vi "Get Value.vi"(10 "Key":string, 11 "Object Entry in":refnum<class "Section.lvclass">) -> (1 "Found?":bool, 2 "Value":refnum<class "Value.lvclass">, 3 "Object Entry out":refnum<class "Section.lvclass">)   [LabVIEW 2024, in "Electronic Datasheet.lvlib" / "Section.lvclass"]
uses:
  Section.lvclass
  Value/Value.lvclass
  Section.lvclass/Section.ctl
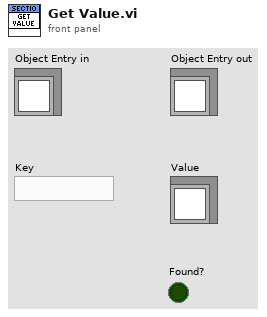
[diagram p1: front panel]
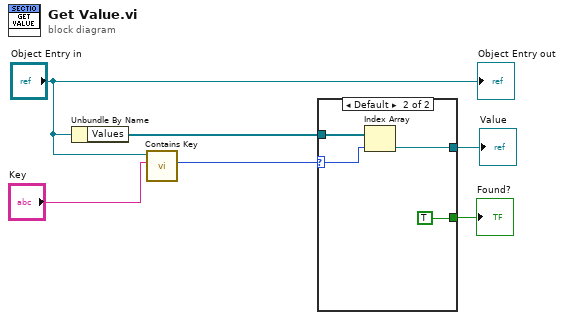
[diagram p0: block diagram]
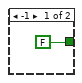
[diagram p2: hidden frame]
diagram:
  n1 = Unbundle By Name("Object Entry in") -> ("Values"=w6:refnum<class "Value.lvclass">[])
  n2 = call "Contains Key.vi"("Key"="Key", "Section in"="Object Entry in") -> ("Index"=w2:i32)  [unwired: 7 in, 2 out]
  n3 = case shown="Default" w2 {
    selector: w2 -> [_ w10]
    tunnel: w6 -> [_ w11]
    tunnel: [_ w9] -> w1
    tunnel: [FALSE TRUE] -> w5
    frame -1 {
    }
    frame Default {
      n4 = Index Array(array=w11, index=w10) -> (element=w9:refnum<class "Value.lvclass">)
    }
  }
  "Found?" <- w5
  "Value" <- w1
  "Object Entry out" <- "Object Entry in"
